vi "Package Typed Message.vi"(8 "error in (no error)":errorcluster, 11 "StringGroup in":refnum<class "StringGroup.lvclass">) -> (0 "error out":errorcluster, 2 "Data Msg":refnum<class "Message.lvclass">, 3 "StringGroup out":refnum<class "StringGroup.lvclass">)   [LabVIEW 2020, in "Vecto.lvlib" / "StringGroup.lvclass"]
uses:
  StringGroup.lvclass
  C:/dev/lv20CE/relink/lv-vecto/Vecto/GroupAbstract/GroupAbstract.lvclass
  lv-protoc/LV-Proto/Message/Message.lvclass
  proto/StringData/Data.ctl
  GroupAbstract/GroupAbstract.lvclass/GroupAbstract.ctl
  Group Config/Group Config.lvclass/Group Config.ctl
  StringGroup.lvclass/StringGroup.ctl
  proto/StringData/Class/Msg.lvclass/Msg.ctl
  proto/StringData/Class/Msg.lvclass
  C:/dev/lv20CE/relink/lv-protoc/LV-Proto/Message/Message.lvclass
  GroupAbstract/GroupAbstract.lvclass
  Group Config/Group Config.lvclass
  proto/StringData/StringData.lvlib
  Vecto.lvlib
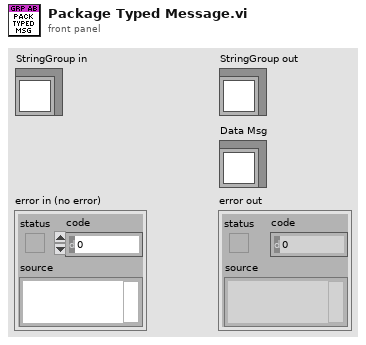
[diagram p1: front panel]
types:
  T1 = typedef "StringData.lvlib/Data.ctl" = cluster{"group_name":string, "data_timestamp":i64, "strings":string[]}
  T2 = typedef "Vecto.lvlib/StringGroup.lvclass/Ref.ctl" = cluster{"Strings":string[], "Timestamp":dbl[]}
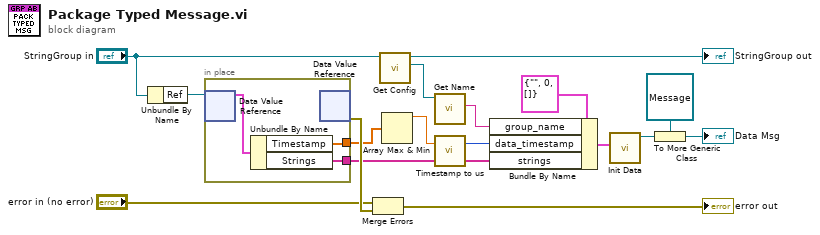
[diagram p0: block diagram]
diagram:
  n1 = Unbundle By Name("StringGroup in") -> ("Ref"=w15:refnum<data-value>)
  n2 = in-place {
    in-place-border: [w19] -> w6
    in-place-border: [w18] -> w13
    n3 = in-place-dvr #1(w15) -> (w20:T2)  [unwired: 1 out]
    n4 = Unbundle By Name(w20) -> ("Timestamp"=w18:dbl[], "Strings"=w19:string[])
    n5 = in-place-dvr #1() -> (w17:errorcluster)  [unwired: 1 in, 1 out]
  }
  n6 = Merge Errors("error in (no error)", w17) -> (→"error out":errorcluster)
  n7 = call "Get Config.vi"("GroupAbstract in"="StringGroup in") -> ("Config"=w11:refnum<class "Group Config.lvclass">, "GroupAbstract out"=→"StringGroup out":refnum<class "StringGroup.lvclass">)  [unwired: 8 in, 1 out]
  n8 = Array Max & Min(array=w13) -> (max value=w7:dbl)  [unwired: 3 out]
  n9 = call "Get Name.vi"("Group Config in"=w11) -> ("Name"=w8:string)  [unwired: 8 in, 2 out]
  n10 = call "Timestamp to us.vi"("Timestamp"=w7) -> ("Timestamp us"=w9:i64)  [unwired: 6 in]
  n11 = Bundle By Name(cluster=T1 {"group_name"="", "data_timestamp"=0, "strings"=[]} ("StringData"), "group_name"=w8, "data_timestamp"=w9, "strings"=w6) -> (w5:T1)
  n12 = call "Init Data.vi"("Data"=w5) -> ("Msg out"=w3:refnum<class "Msg.lvclass">)  [unwired: 10 in]
  n13 = To More Generic Class(target class=refnum<class "Message.lvclass"> refnum ("LV-Proto.lvlib:Message.lvclass"), reference=w3) -> (generic class reference=→"Data Msg":refnum<class "Message.lvclass">)
